vi "Use Custom Object Menu.vi"(8 "Error In":errorcluster, 10 "Menu in":refnum<k9>, 11 "CtlRef":refnum<vi>) -> (0 "error out":errorcluster, 2 "Menu out":refnum<k9>, 3 "CtlRef dup":refnum<vi>)   [LabVIEW 2019]
uses:
  Edit Object's Custom Run-Time Right-Click Menu.llb/Menu Description.ctl
  <vilib>/UserTags/UserTags.lvlib
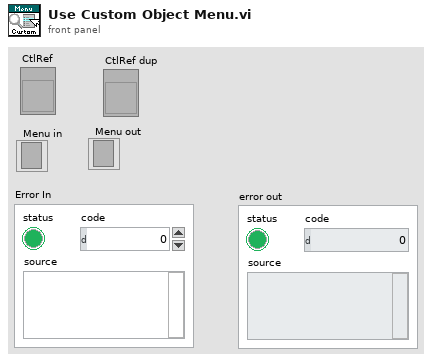
[diagram p1: front panel]
types:
  T1 = typedef "Menu Description.ctl" = cluster{"Item Descriptions":string[][], "Used Items":bool[]}
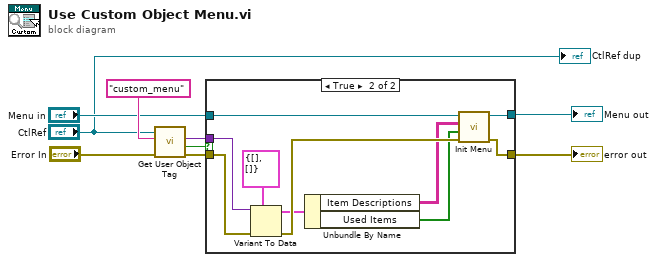
[diagram p0: block diagram]
diagram:
  n1 = call <vilib>:"Get User Object Tag.vi"("error in (no error)"="Error In", "Tag Name"="custom_menu", "Generic Refnum"="CtlRef") -> ("error out"=w5:errorcluster, "Was Tag Found?"=w7:bool, "Value"=w6:variant)  [unwired: 5 in, 1 out]
  n2 = case shown="True" w7 {
    tunnel: "Menu in" -> [w11 w21]
    tunnel: w5 -> [w10 w15]
    tunnel: w6 -> [_ w14]
    tunnel: [w11 w13] -> w8
    tunnel: [w10 w12] -> w9
    frame False {
    }
    frame True {
      n3 = Variant To Data(error in=w15, type=T1 {"Item Descriptions"=[], "Used Items"=[]} ("Menu Description"), Variant=w14) -> (data=w18:T1, error out=w19:errorcluster)
      n4 = Unbundle By Name(w18) -> ("Item Descriptions"=w17:string[][], "Used Items"=w16:bool[])
      n5 = call "Init Menu.vi"("Error In"=w19, "Used Items"=w16, "Item Names"=w17, "Menu in"=w21) -> ("Error Out"=w12:errorcluster, "menu reference out"=w13:refnum<k9>)  [unwired: 6 in]
    }
  }
  "error out" <- w9
  "Menu out" <- w8
  "CtlRef dup" <- "CtlRef"
